vi "ZControlSolenoid - Copy.vi"() -> ()   [LabVIEW 2014]
uses:
  <vilib>/DAQmx/write.llb/DAQmx Write (Digital 1D Bool NChan 1Samp 1Line).vi
panel:
  in  "On?":bool
  in  "stop":bool
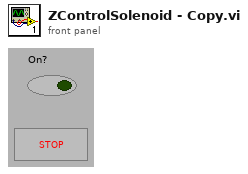
[diagram p1: front panel]
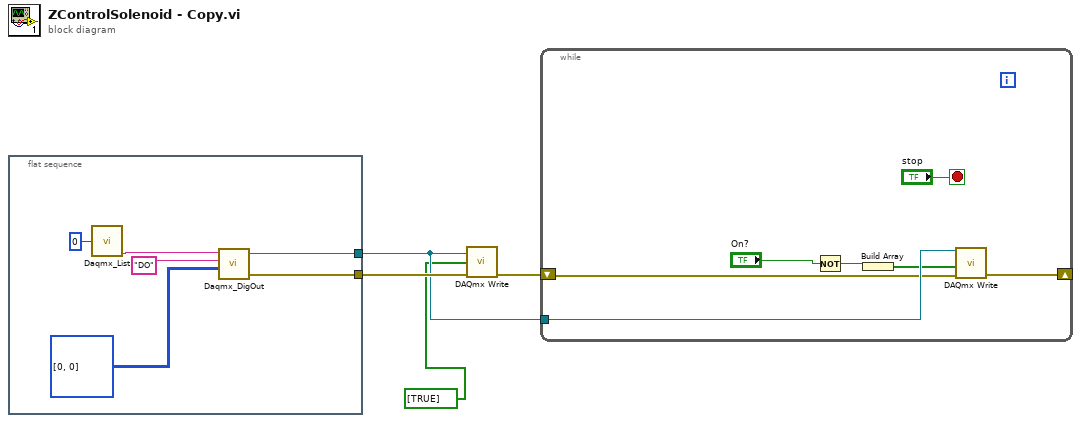
[diagram p0: block diagram]
diagram:
  n1 = flat-sequence {
    tunnel: [w6] -> w4
    tunnel: [w7] -> w2
    frame #0 {
      n2 = call "Daqmx_List.vi"("Device Number n"=u8 0) -> ("NI-DAQmx Device Name n"=w8:tag)  [unwired: 3 out]
      n3 = call "Daqmx_DigOut.vi"("Array of Ports, Lines"=u8[][] [[0, 0]], "Base Task Name"="DO", "DAQmx device name"=w8) -> ("error out"=w6:errorcluster, "Output Task Name"=w7:refnum<k21>)  [unwired: 1 in, 1 out]
    }
  }
  n4 = call-poly <vilib>:"DAQmx Write.vi"("task/channels in"=w2, "data"=bool[] [TRUE], "error in"=w4) -> ("error out"=w3:errorcluster)  [unwired: 1 in, 11 out]
  n5 = while {
    tunnel: w2 -> [w16]
    shift-right: [w15] -> _
    shift-left: w3 -> [w13]
    stop <- "stop" stop-if-true
    n6 = Not(x="On?") -> (.not. x?=w12:bool)
    n7 = Build Array(w12) -> (w11:bool[])
    n8 = call-poly <vilib>:"DAQmx Write.vi"("task/channels in"=w16, "data"=w11, "error in"=w13) -> ("error out"=w15:errorcluster)  [unwired: 1 in, 11 out]
  }
